vi "armcontrol.vi"   [LabVIEW 2012, in "BlockParty4150.lvrbt"]
uses:
  BlockParty4150.lvrbt
  <vilib>/NXT/Block Support/NXT_ButtonSelector.ctl
  <vilib>/NXT/Hardware/Plugins/Tetrix DC Motor/TetrixDCMotorAddress.ctl
  <vilib>/NXT/NXTIO Xnodes/NXTIONodeSubVIs/TETRIX IO Move DC Motors.vi
  <vilib>/NXT/Subs/LVHSConnector.ctl
  <vilib>/NXT/NXTIO Xnodes/AddressXNode/NXTIOAddress.xnode
  <vilib>/NXT/NXTIO Xnodes/NXTIOXNode/NXTIO.xnode
  <vilib>/NXT/LegoClasses/BrickReference/BrickReference.lvclass
types:
  T1 = typedef "TetrixDCMotorAddress.ctl" = i16
  T2 = cluster{"TetrixDCMotor":T1, "TetrixDCMotor 2":T1}
  T3 = typedef "NXT_ButtonSelector.ctl" = u16
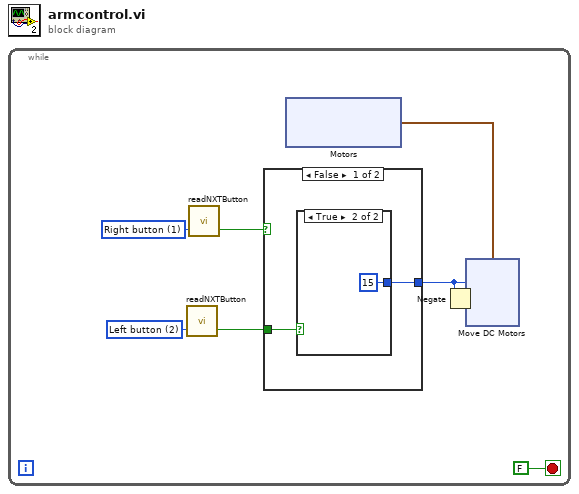
[diagram p0: block diagram]
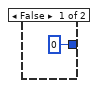
[diagram p2: hidden frame]
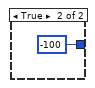
[diagram p3: hidden frame]
diagram:
  n1 = while {
    stop <- FALSE stop-if-true
    w6 = T3 1 items=["Enter button"=3, "Left button"=2, "Right button"=1] ("Button (Enter button)")
    w7 = T3 2 items=["Enter button"=3, "Left button"=2, "Right button"=1] ("Button (Enter button)")
    n2 = call <vilib>:"readNXTButton.vi"("Button (Enter button)"=w7) -> ("Yes/No"=w4:bool)  [unwired: 2 in, 1 out]
    n3 = call <vilib>:"readNXTButton.vi"("Button (Enter button)"=w6) -> ("Yes/No"=w5:bool)  [unwired: 2 in, 1 out]
    n4 = case shown="False" w5 {
      tunnel: w4 -> [w21 _]
      tunnel: [w20 i8 -100 ("Power/Speed 1")] -> w2
      frame False {
        n5 = case shown="True" w21 {
          tunnel: [i8 0 ("Power/Speed 1") i8 15 ("Power/Speed 1")] -> w20
          frame False {
          }
          frame True {
          }
        }
      }
      frame True {
      }
    }
    n6 = xnode "Motors"() -> ("Motor"=w3:cluster{"TetrixDCMotor":T1, "TetrixDCMotor":T1})
    n7 = Negate(x=w2) -> (-x=w1:i8)
    n8 = xnode "Move DC Motors"("Power/Speed 2"=w1, "Power/Speed 1"=w2, "Motors"=w3) -> ()  [unwired: 1 in, 1 out]
  }
